vi "Read Local Resource.vi"(8 "error in (no error)":errorcluster, 11 "69X_79X In":refnum<class "7976A.lvclass">) -> (0 "error out":errorcluster, 2 "Local Resource":refnum<visa-resource-name>, 3 "69X_79X Out":refnum<class "7976A.lvclass">)   [LabVIEW 2019, in "7976A.lvlib" / "7976A.lvclass"]
uses:
  Library/7976A.lvclass
  Library/7976A.lvclass/7976A.ctl
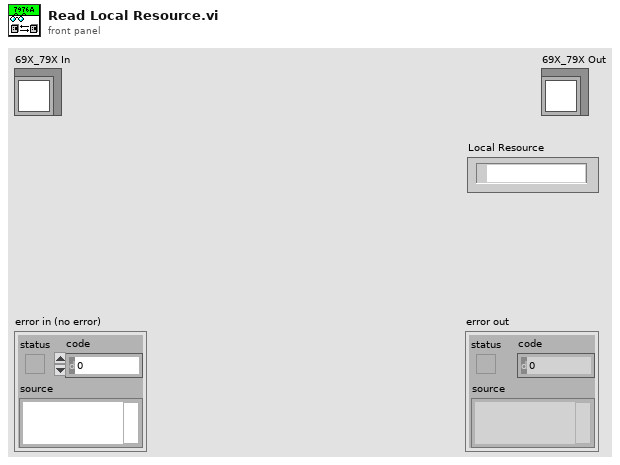
[diagram p1: front panel]
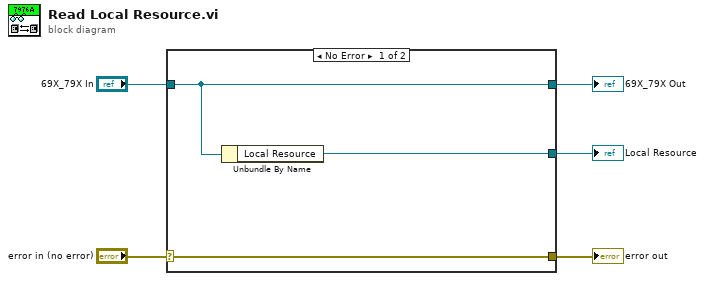
[diagram p0: block diagram]
diagram:
  n1 = case shown="No Error" "error in (no error)" {
    selector: "error in (no error)" -> [w8 w9]
    tunnel: [w8 w9] -> w5
    tunnel: [w7 w10] -> w2
    tunnel: "69X_79X In" -> [w7 w10]
    tunnel: [w6 _] -> w1
    frame No Error {
      n2 = Unbundle By Name(w7) -> ("Local Resource"=w6:refnum<visa-resource-name>)
    }
    frame Error {
    }
  }
  "Local Resource" <- w1
  "error out" <- w5
  "69X_79X Out" <- w2
